vi "TestStand - Create Test Data Cluster.vi"(1 "Report Text":string, 2 "String Measurement":string, 3 "Numeric Measurement":dbl format="%.2f", 4 "PASS/FAIL Flag":bool) -> (0 "Test Data":T1 {"Numeric Measurement" format="%.2f"})   [LabVIEW 2012]
doc: "Bundles together the data necessary to create the Test Data cluster that the TestStand LabVIEW Standard Prototype Adapter requires on test VIs."
uses:
  LabVIEW Test - Test Data.ctl
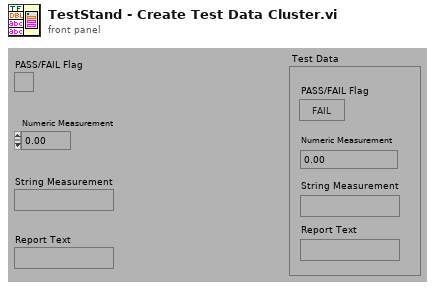
[diagram p1: front panel]
types:
  T1 = typedef "LabVIEW Test - Test Data.ctl" = cluster{"PASS/FAIL Flag":bool, "Numeric Measurement":dbl, "String Measurement":string, "Report Text":string}
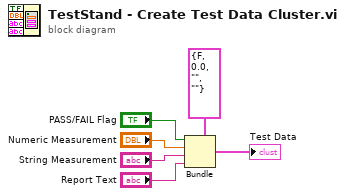
[diagram p0: block diagram]
diagram:
  n1 = Bundle(cluster=T1 {"PASS/FAIL Flag"=FALSE, "Numeric Measurement"=0.0, "String Measurement"="", "Report Text"=""} ("Test Data"), "PASS/FAIL Flag"="PASS/FAIL Flag", "Numeric Measurement"="Numeric Measurement", "String Measurement"="String Measurement", "Report Text"="Report Text") -> (→"Test Data":T1)
